vi "DAQ_fileAnalog_Data.vi"() -> ()   [LabVIEW 2020]
uses:
  <vilib>/express/express analysis/Spectral/Block/exnSpectralBlock spectral measurements RMS poly.vi
  <vilib>/express/express analysis/Spectral/Block/exnSpectralBlock spectral measurements RMS DDT.vi
  <vilib>/express/express analysis/Spectral/XNode/ExpressSpectralMeasurementsBlockNode.xnode
panel:
  out "LED ON <1.5 V":bool
  out "PHASE FFT":dynamicdata(graph)
  out "frequenct FFT":dynamicdata(graph)
  out "Amplitude":dynamicdata(graph)
  out "Frequency":dynamicdata(graph)
  out "arbitary signal":dynamicdata(graph) caption="data"
  out "Filtered Signal":dynamicdata(graph)
  out "Tested Signals":dynamicdata(graph)
  in  "stop":bool
  out "data":dbl
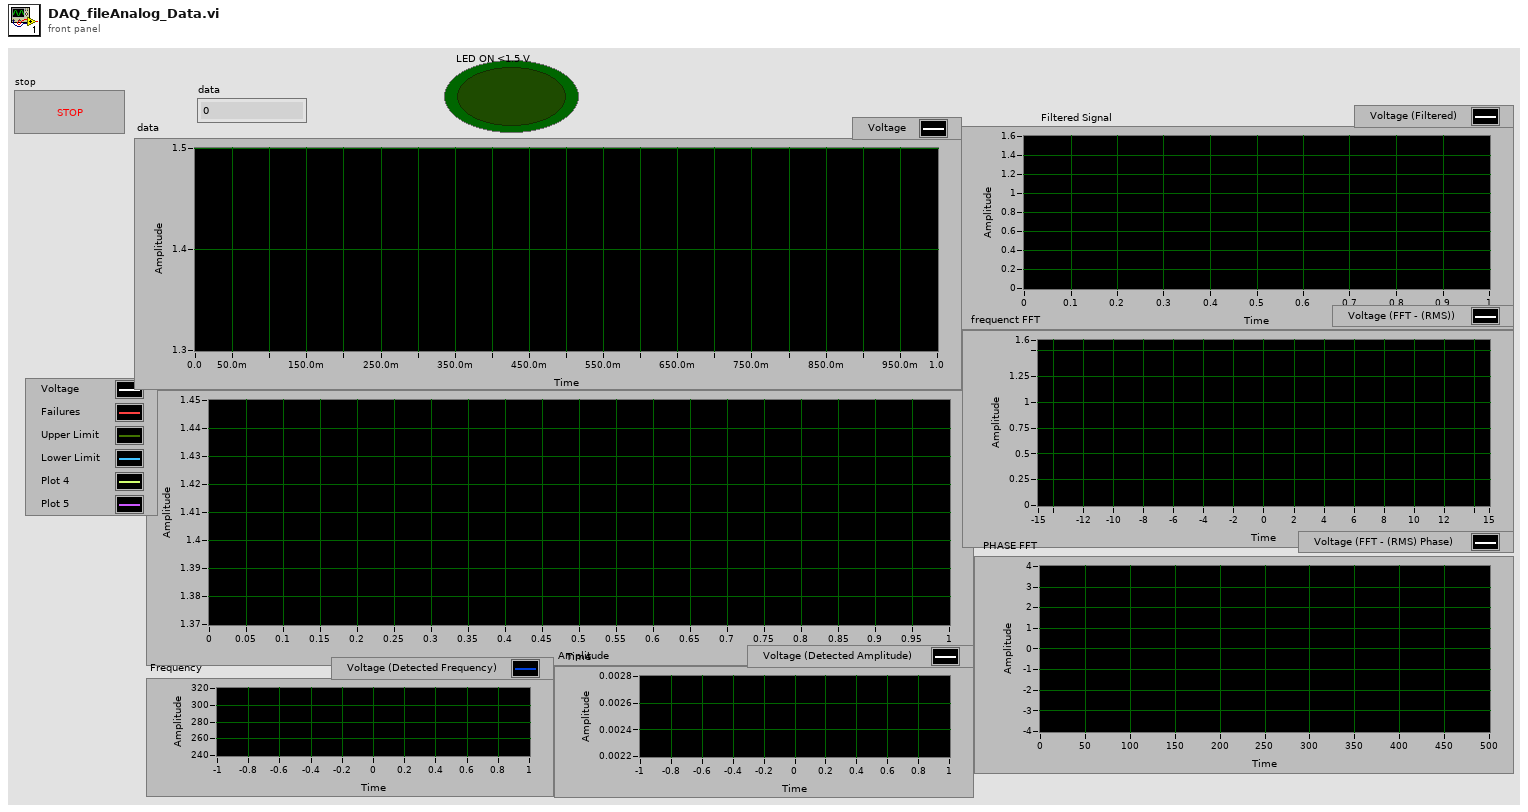
[diagram p1: front panel]
types:
  T1 = cluster{"averaging mode":u16, "weighting mode":u16, "number of averages":u32}
  T2 = cluster{"dB On (F)":bool, "unwrap phase (F)":bool, "convert to degree (F)":bool}
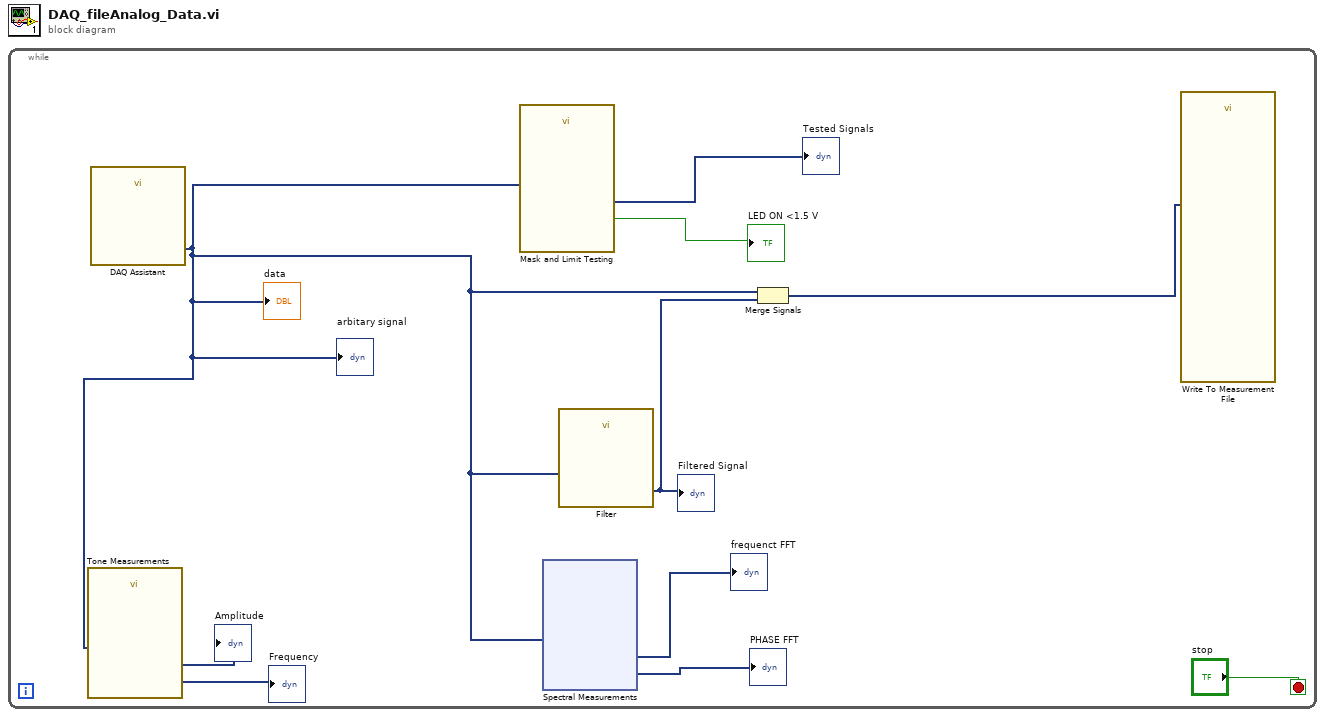
[diagram p0: block diagram]
diagram:
  n1 = while {
    stop <- "stop" stop-if-true
    n2 = call "DAQ Assistant"() -> ("data"=w6:dynamicdata)  [unwired: 17 in, 2 out]
    "data" <- w6
    "arbitary signal" <- w6
    n3 = call "Tone Measurements"("Signals"=w6) -> ("Frequency"=→"Frequency":dynamicdata, "Amplitude"=→"Amplitude":dynamicdata)  [unwired: 8 in, 1 out]
    n4 = call "Mask and Limit Testing"("Signals"=w6) -> ("Passed"=→"LED ON <1.5 V":bool, "Tested Signals"=→"Tested Signals":dynamicdata)  [unwired: 7 in, 2 out]
    n5 = xnode "Spectral Measurements"("Signals"=w6) -> ("FFT - (RMS)"=→"frequenct FFT":dynamicdata, "Phase"=→"PHASE FFT":dynamicdata)  [unwired: 1 in, 1 out]
    n6 = call "Filter"("Signal"=w6) -> ("Filtered Signal"=w2:dynamicdata)  [unwired: 9 in, 1 out]
    "Filtered Signal" <- w2
    n7 = Merge Signals(w6, w2) -> (w3:dynamicdata)
    n8 = call "Write To Measurement File"("Signals"=w3) -> ()  [unwired: 16 in, 3 out]
  }
